vi "Dispose NotifyIcon Refernece.vi"(8 "error in (no error)":errorcluster, 11 "reference":T1) -> (0 "error out":errorcluster)   [LabVIEW 2019, in "Test Bench Tools.lvlib"]
uses:
  Test Bench Tools.lvlib
  System.Windows.Forms
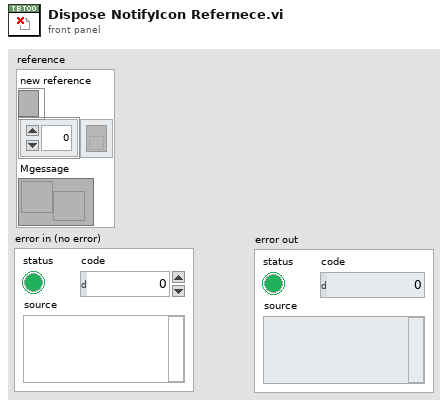
[diagram p1: front panel]
types:
  T1 = cluster{"new reference":refnum<k24>, "Array":refnum<k27>[], "Mgessage":refnum<user-event>}
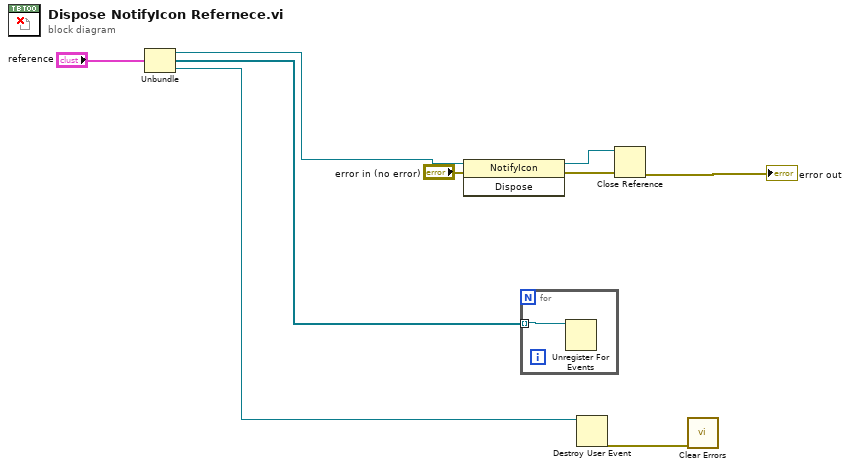
[diagram p0: block diagram]
diagram:
  n1 = Unbundle("reference") -> ("new reference"=w4:refnum<k24>, "Array"=w5:refnum<k27>[], "Mgessage"=w2:refnum<user-event>)
  n2 = invoke class="NotifyIcon" method="Dispose"(reference=w4, error in="error in (no error)") -> (reference out=w9:refnum<k24>, error out=w8:errorcluster)  [unwired: 1 in, 1 out]
  n3 = for {
    tunnel: w5 -> [w10] mode=indexing
    n4 = Unregister For Events(event registration refnum=w10) -> ()  [unwired: 1 in, 1 out]
  }
  n5 = Destroy User Event(user event=w2) -> (error out=w1:errorcluster)  [unwired: 1 in]
  n6 = Close Reference(reference=w9, error in (no error)=w8) -> (error out=→"error out":errorcluster)
  n7 = call <vilib>:"Clear Errors.vi"("error in (no error)"=w1) -> ()  [unwired: 5 in, 2 out]
